vi "Start Secure TCP.vi"(8 "error in (no error)":errorcluster, 11 "Server in":refnum<class "Server.lvclass">) -> (0 "error out":errorcluster, 3 "Server out":refnum<class "Server.lvclass">)   [LabVIEW 2020, in "HTTP Server.lvlib" / "Server.lvclass"]
uses:
  Server.lvclass
  Server.lvclass/Server.ctl
  lv-uri/URI/URI/URI.lvclass
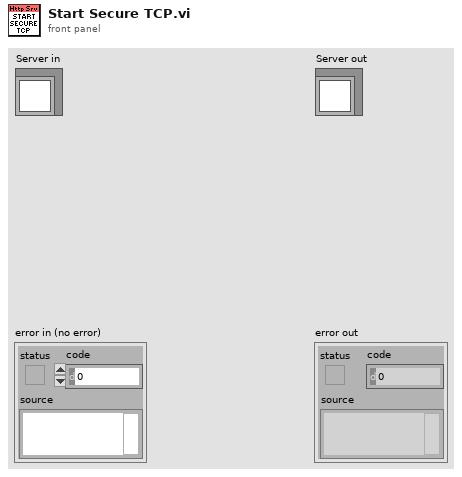
[diagram p1: front panel]
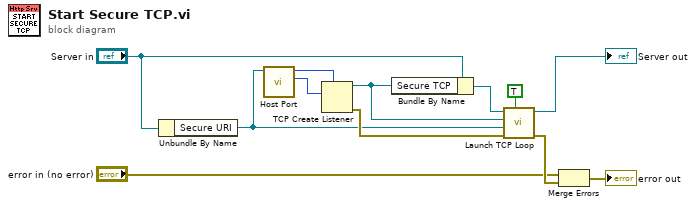
[diagram p0: block diagram]
diagram:
  n1 = Unbundle By Name("Server in") -> ("Secure URI"=w8:refnum<class "URI.lvclass">)
  n2 = call "Host Port.vi"("URI in"=w8) -> ("Port"=w10:u16, "Host"=w11:u32)  [unwired: 8 in, 1 out]
  n3 = TCP Create Listener(7:w11, 10:w10) -> (0:w12:errorcluster, 3:w9:refnum<k5>)  [unwired: 3 in, 1 out]
  n4 = Bundle By Name(cluster="Server in", "Secure TCP"=w9) -> (w5:refnum<class "Server.lvclass">)
  n5 = call "Launch TCP Loop.vi"("Secure"=TRUE, "error in (no error)"=w12, "Server URI"=w8, "TCP"=w9, "Server in"=w5) -> ("error out"=w6:errorcluster, "Server out"=→"Server out":refnum<class "Server.lvclass">)  [unwired: 5 in]
  n6 = Merge Errors("error in (no error)", w6) -> (→"error out":errorcluster)
